vi "RIB Req - eSTOP 1.vi"(0 "Limits File Path":path, 5 "Results File Path":path, 11 "error in":errorcluster) -> (4 "Results Data Array":string[][](array[string]), 15 "error out":errorcluster)   [LabVIEW 2024]
doc: "Template test"
uses:
  <vilib>/addons/_JKI Toolkits/State Machine/_JKI_lib_State_Machine.llb/Select State(s)_err__jki_lib_state_machine.vi
  <vilib>/addons/_JKI Toolkits/State Machine/_JKI_lib_State_Machine.llb/Select State(s)_bool__jki_lib_state_machine.vi
  <vilib>/addons/_JKI Toolkits/State Machine/_JKI_lib_State_Machine.llb/Periodic Trigger__ogtk__JKI-SM__jki_lib_state_machine.vi
  <userlib>/_OpenG.lib/file/file.llb/Strip Path Extension - String__ogtk.vi
  <vilib>/Utility/file.llb/Read Delimited Spreadsheet (string).vi
  <userlib>/_OpenG.lib/file/file.llb/openg_file.lvlib
  <userlib>/_OpenG.lib/appcontrol/appcontrol.llb/openg_application_control.lvlib
  <userlib>/_OpenG.lib/time/time.llb/openg_time.lvlib
  <vilib>/Utility/file.llb/Write Delimited Spreadsheet (string).vi
panel:
  out "Wait for Start":bool
  out "Normal Operation":bool
  out "Wait - Reset":u32(slide)=1 scale=0.0..10.0
  in  "eSTOP 1 State Error Test":string
  in  "eSTOP 1 State Test":string
  in  "Read Start":string
  in  "Read Set":string
  out "Timeout - Error Test":dbl(slide) scale=0.0..3.0
  out "Timeout - Test":dbl(slide) scale=0.0..3.0
  out "eSTOP 1 Test":bool
  out "eSTOP 1 Error Test":bool
  in  "eSTOP 1 Error Test":string
  in  "eSTOP 1 Test":string
  in  "connection ID":refnum<k16>
  in  "handle out":u64
  in  "Exit":bool
  # "eSTOP 1 Test"
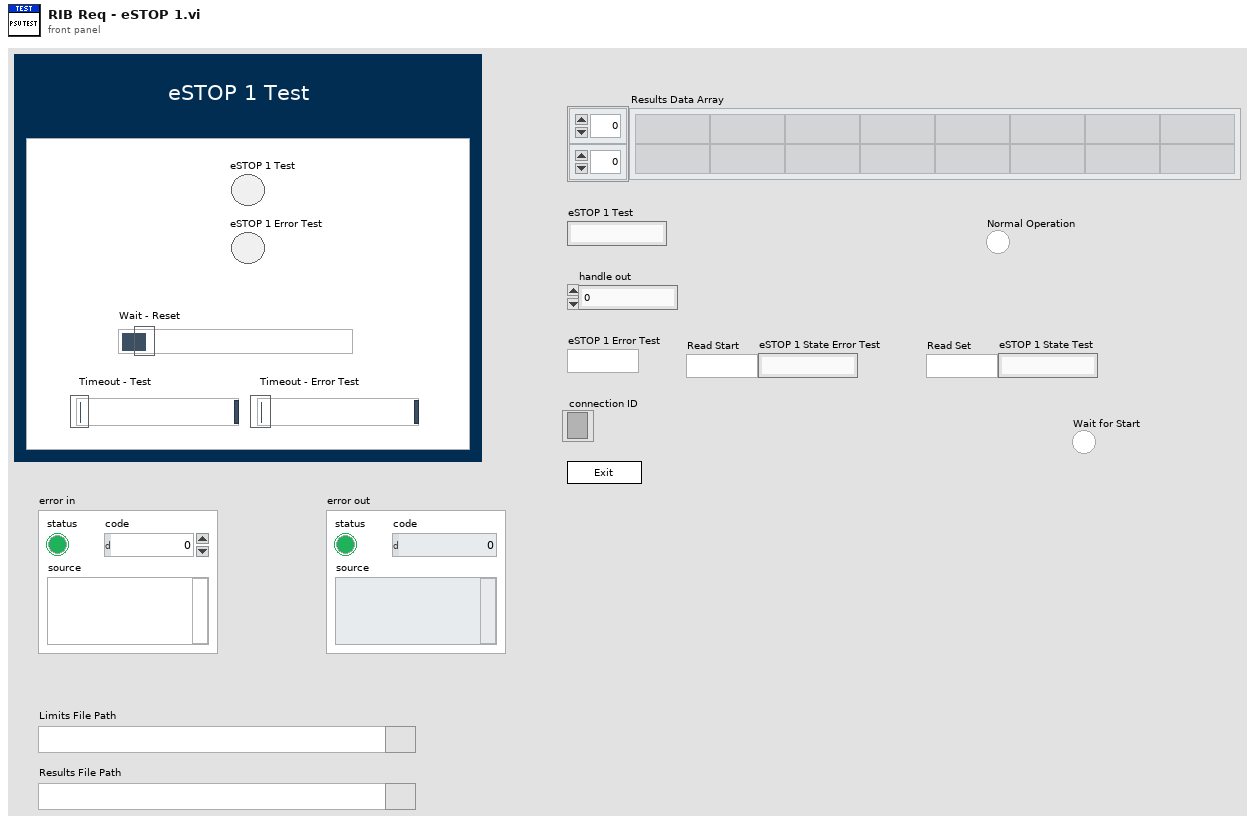
[diagram p1: front panel]
types:
  T1 = enum32{"Invalid", "Standard", "Closed", "Hidden", "Minimized", "Maximized"}
  T2 = enum32{"invalid app kind", "Development System", "Run Time System", "Student Edition", "Embedded LabVIEW", "Evaluation", "Custom"}
  T3 = typedef "FGV - Enum" = enum16{"Cleanup", "Get Data", "Open UDP", "Initialise DAQ", "Initialise I2C"}
  T4 = enum16{"Start Timer", "Get Time", "Pause", "Unpause"}
  T5 = cluster{"Core":cluster{"Current VI Reference":refnum<vi>, "Close Panel on Exit?":bool}, "Limits File Path":path, "Test Limits":string[][], "Results Data Array":string[][], "Results File Path":path, "Voltage":dbl, "connection ID":refnum<k16>, "handle out":u64, "eSTOP 1 Test":string, "eSTOP 1 Error Test":string, "Read Set":string, "Read Start ":string, "eSTOP 1 State Test":string, "eSTOP 1 State Error Test":string}
  T6 = cluster{"Current VI Reference":refnum<vi>, "Close Panel on Exit?":bool}
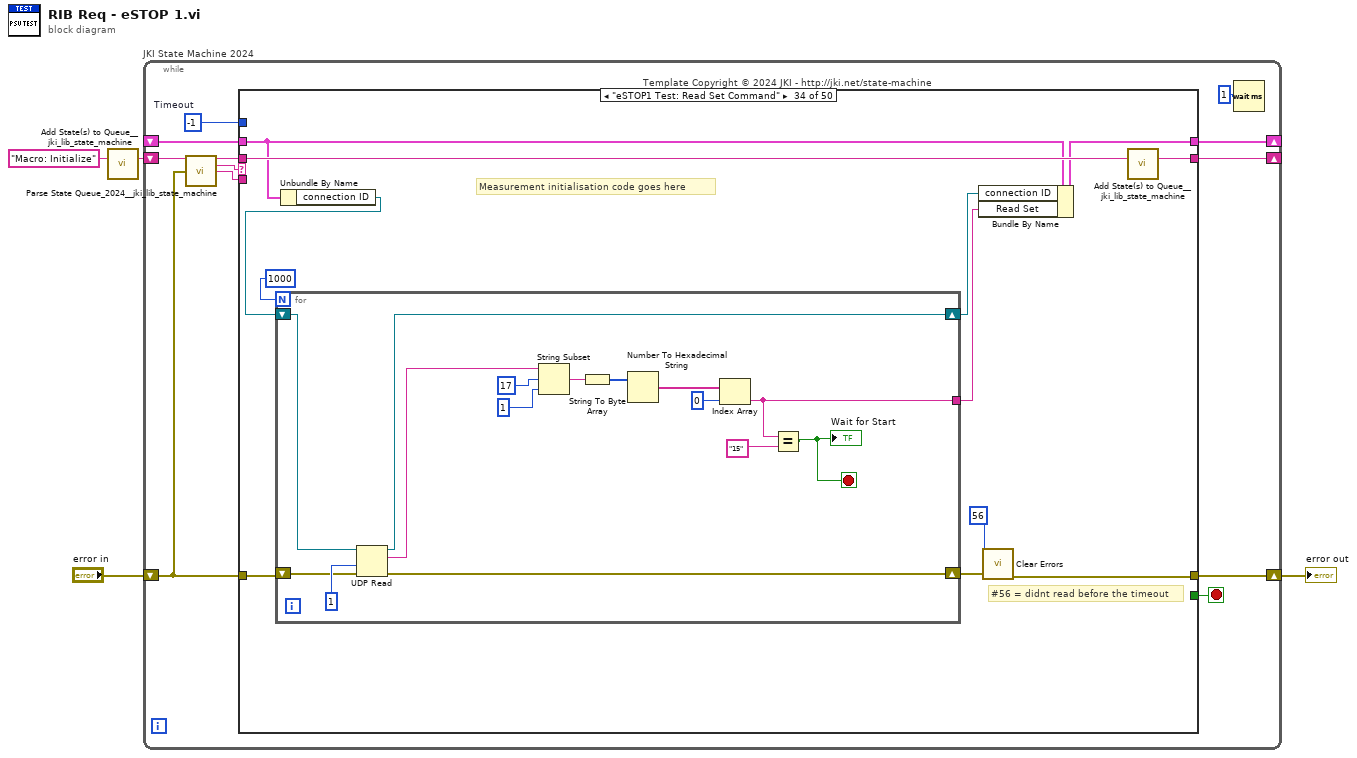
[diagram p0: block diagram]
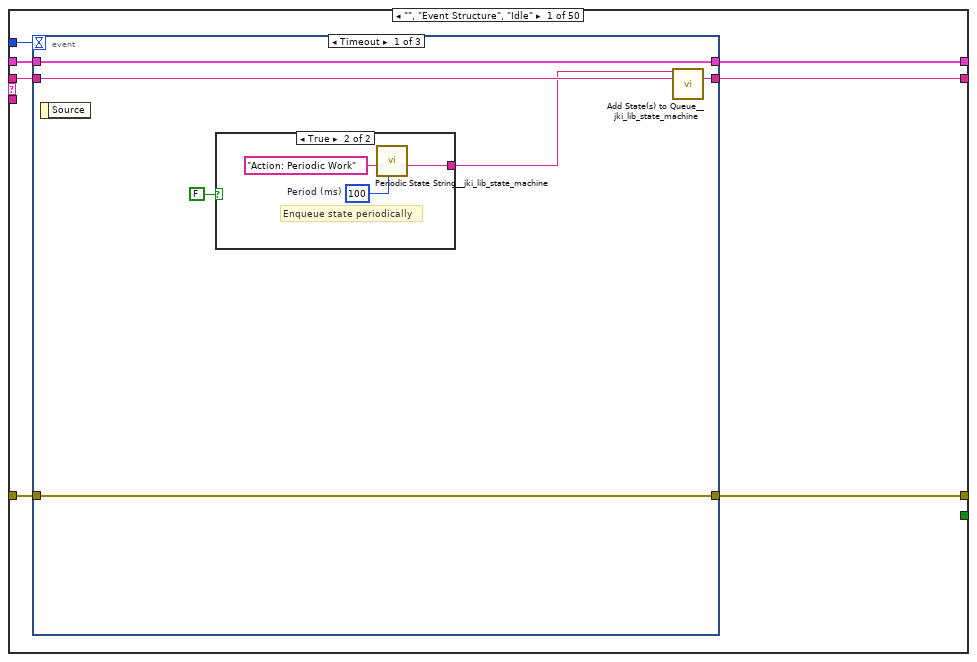
[diagram p2: hidden frame]
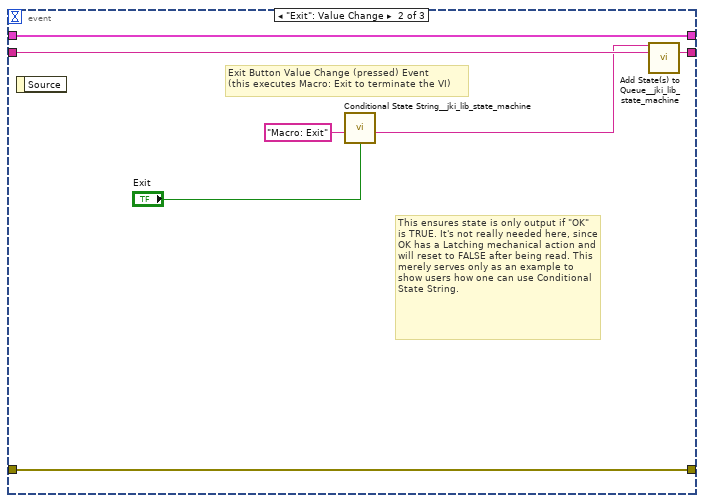
[diagram p4: hidden frame]
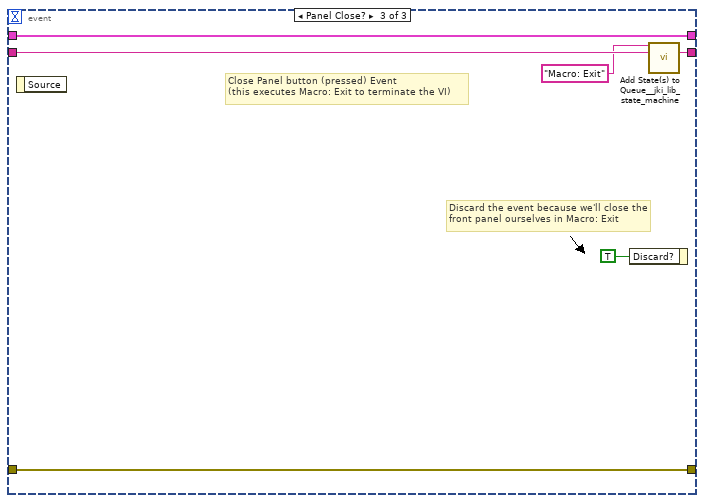
[diagram p5: hidden frame]
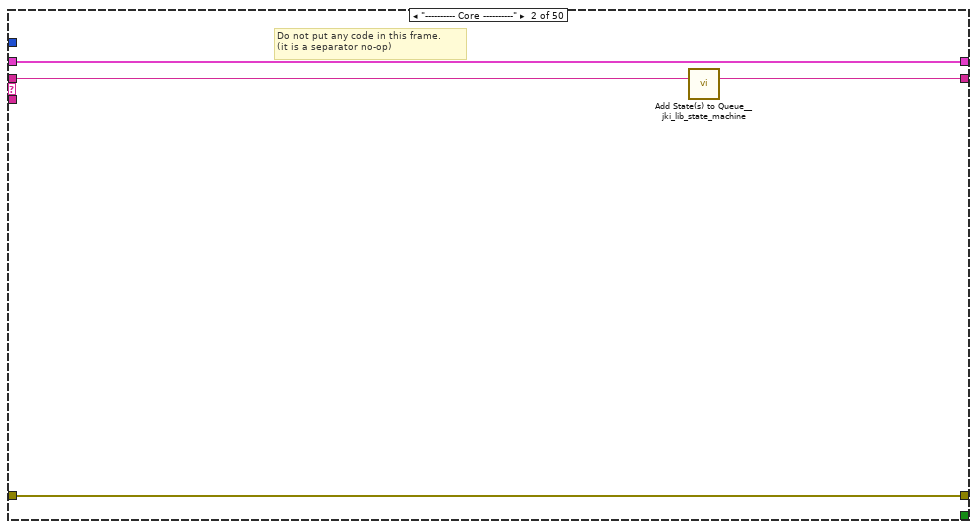
[diagram p6: hidden frame]
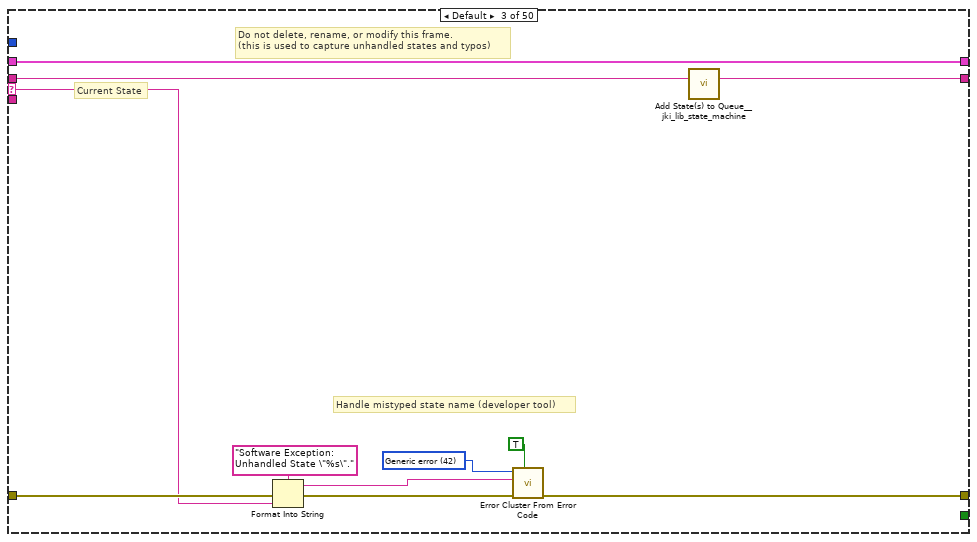
[diagram p7: hidden frame]
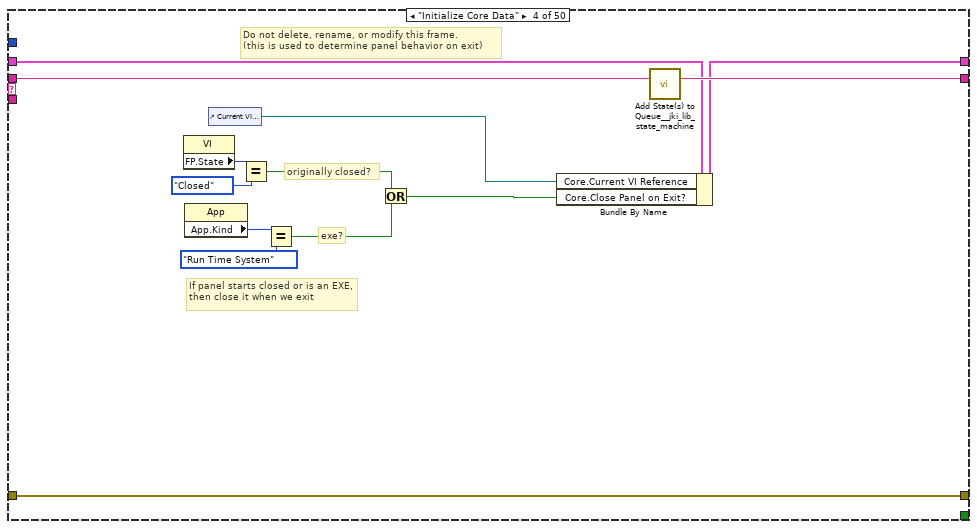
[diagram p8: hidden frame]
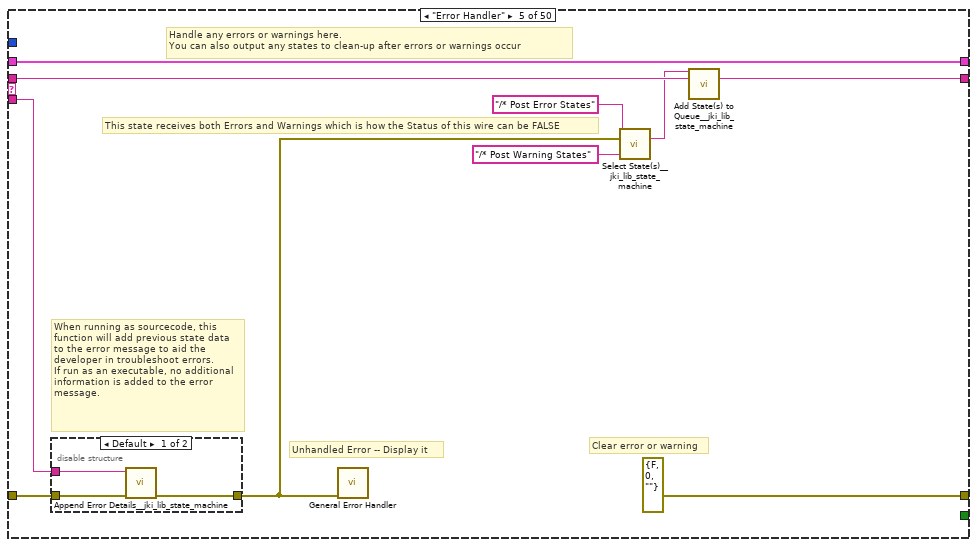
[diagram p9: hidden frame]
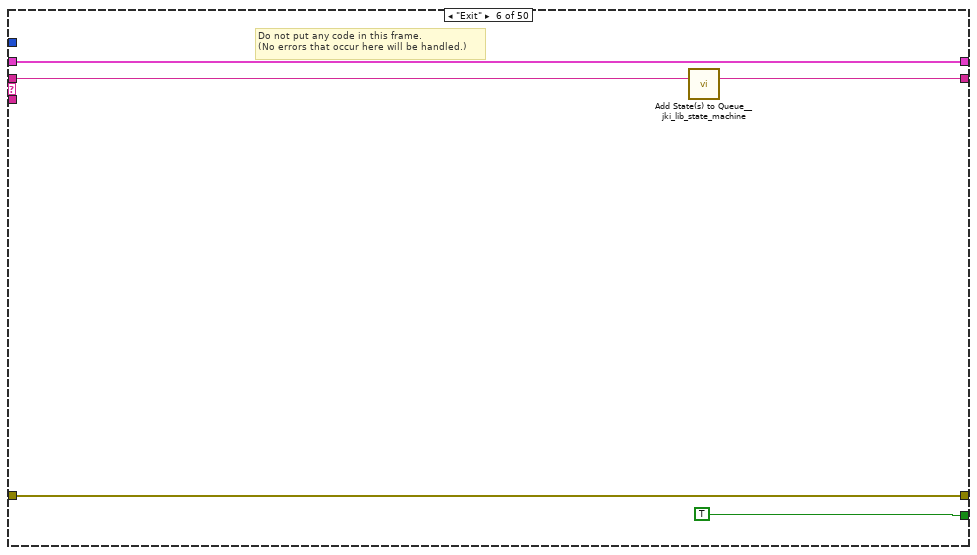
[diagram p11: hidden frame]
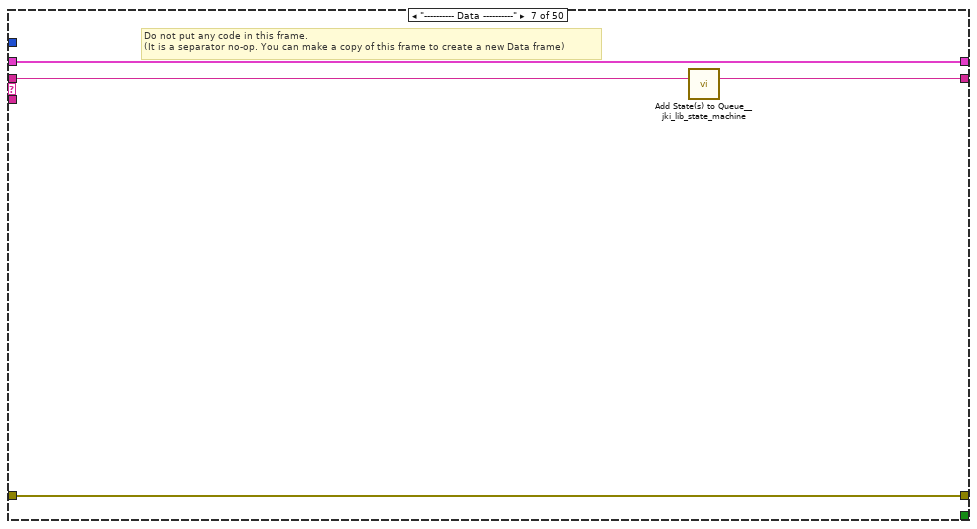
[diagram p12: hidden frame]
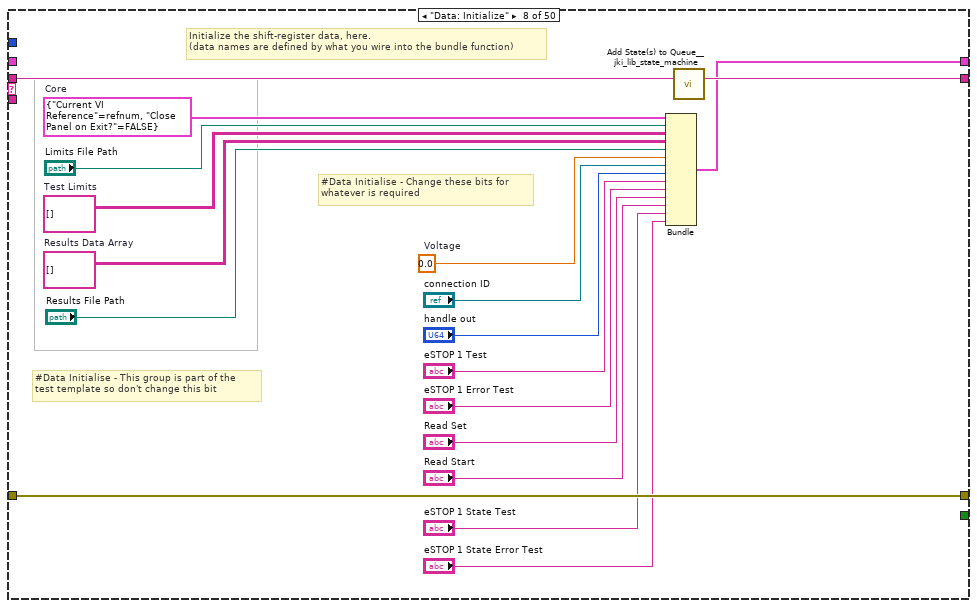
[diagram p13: hidden frame]
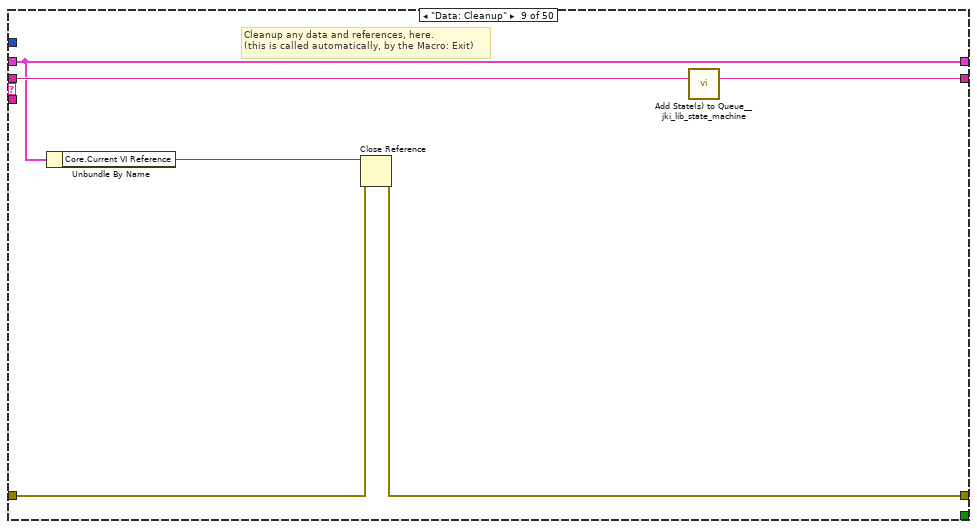
[diagram p14: hidden frame]
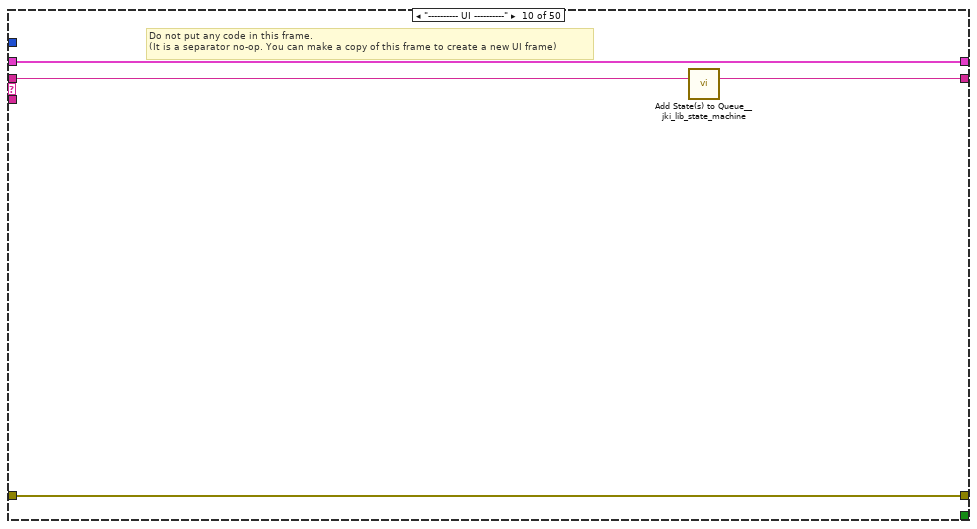
[diagram p15: hidden frame]
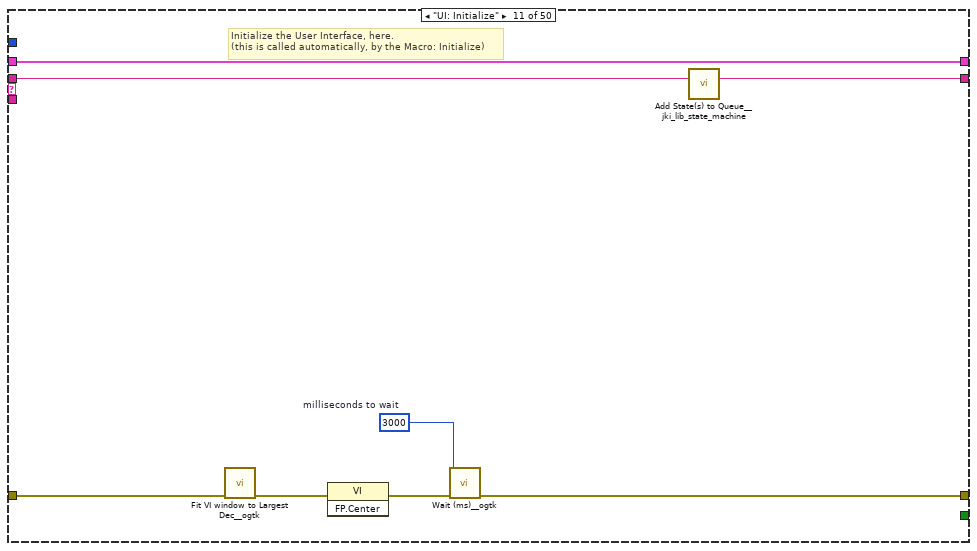
[diagram p16: hidden frame]
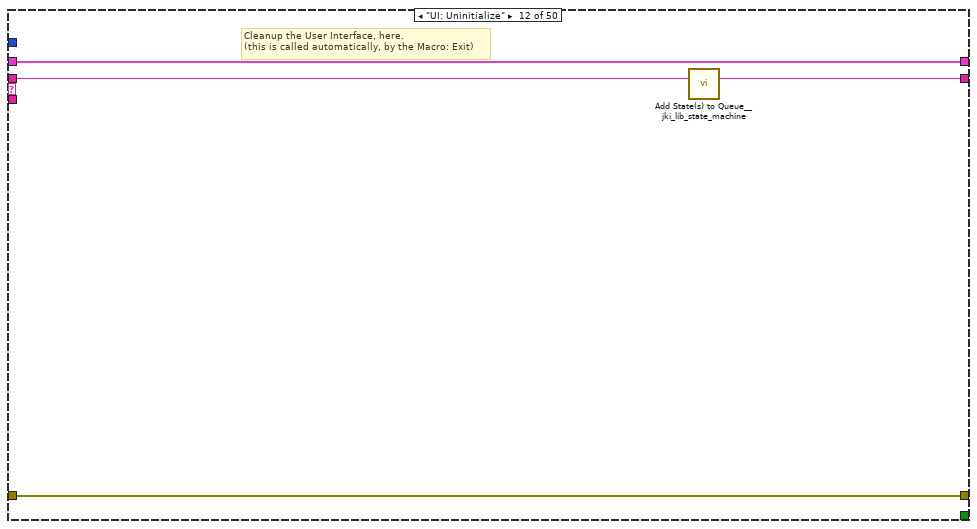
[diagram p17: hidden frame]
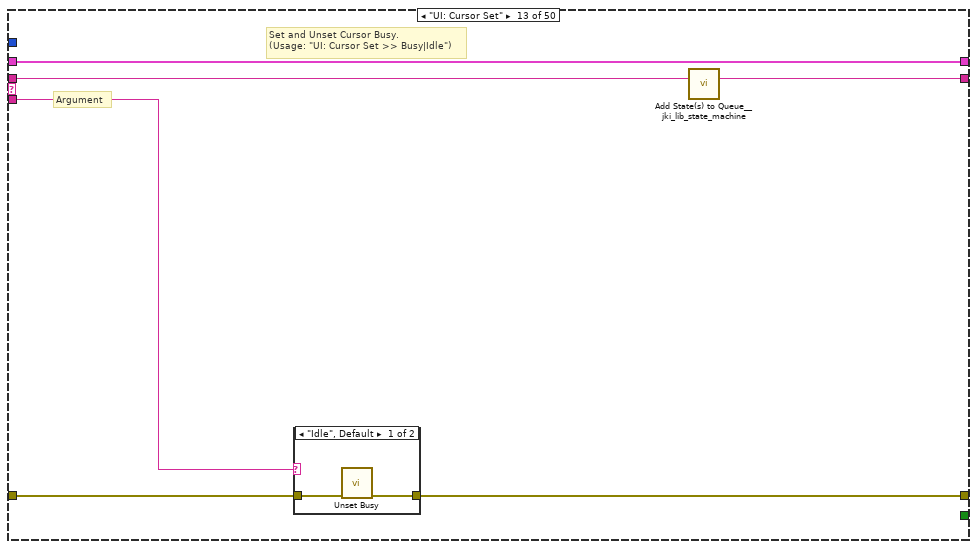
[diagram p18: hidden frame]
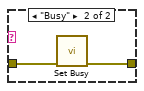
[diagram p19: hidden frame]
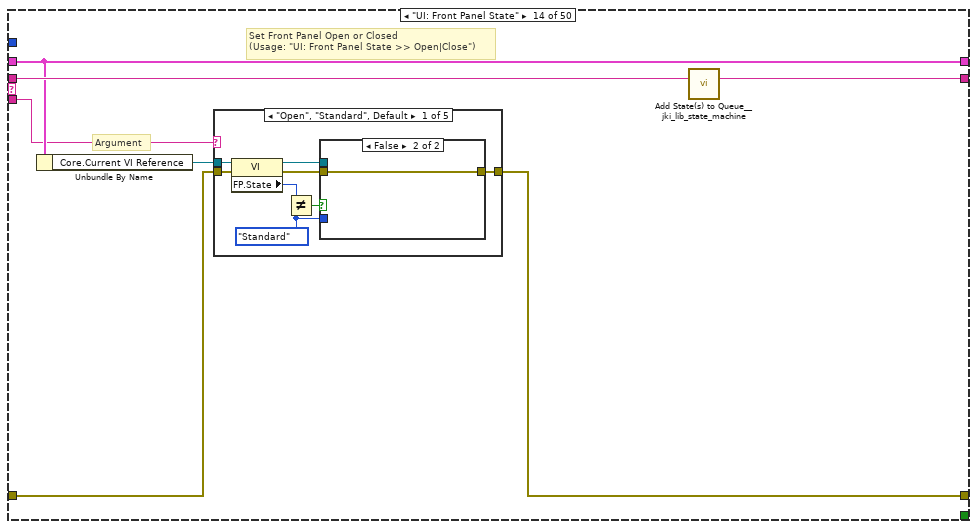
[diagram p20: hidden frame]
diagram:
  n1 = call <vilib>:"Add State(s) to Queue__jki_lib_state_machine.vi"("State(s) in (\"\")"="Macro: Initialize") -> ("States Out"=w4:string)  [unwired: 14 in]
  n2 = while "JKI State Machine 2024" {
    shift-right: [w9] -> _
    shift-left: _ -> [w8]
    shift-right: [w12] -> w1
    shift-left: "error in" -> [w6]
    shift-right: [w11] -> _
    shift-left: w4 -> [w13]
    stop <- w10 stop-if-true
    w7 = -1  # Timeout
    # "Template Copyright © 2024 JKI - http://jki.net/state-machine"
    n3 = call <vilib>:"Parse State Queue_2024__jki_lib_state_machine.vi"("State Queue"=w13, "Error In (no error)"=w6) -> ("Remaining States"=w15:string, "Current State"=w16:string, "Arguments"=w14:string)  [unwired: 11 in]
    n4 = case shown="\"eSTOP1 Test: Read Set Command\"" w16 {
      selector: w16 -> [_ _ w50 _ _ _ _ _ _ _ _ _ _ _ _ _ _ _ _ _ _ _ _ _ _ _ _ _ _ _ _ _ _ _ _ _ _ _ _ _ _ _ _ _ _ _ _ _ _ _]
      tunnel: w15 -> [w23 w49 w54 w73 w83 w92 w96 w114 w120 w124 w132 w136 w142 w153 w222 w227 w232 w237 w242 w251 w255 w268 w285 w298 w311 w324 w337 w350 w354 w363 w367 w376 w397 w409 w445 w457 w482 w491 w515 w539 w551 w560 w582 w603 w614 w624 w648 w672 w684 w693]
      tunnel: w14 -> [_ _ _ _ w78 _ _ _ _ _ _ _ w137 w147 _ _ _ _ _ _ _ _ _ _ _ _ _ _ _ _ _ _ _ _ _ _ _ _ _ _ _ _ _ _ _ _ _ _ _ _]
      tunnel: w8 -> [w21 w46 w52 w66 w80 w90 w93 _ w115 w121 w130 w134 w140 w149 w219 w224 w229 w234 w239 w249 w252 w258 w277 w290 w303 w316 w329 w342 w351 w359 w364 w374 w394 w406 w442 w454 w480 w485 w498 w522 w549 w553 w579 w600 w612 w618 w631 w655 w682 w686]
      tunnel: [w20 w47 w56 w70 errorcluster {"status"=FALSE, "code"=0, "source"=""} ("error out") w89 w94 w111 w116 w122 w128 w133 w138 w150 w220 w225 w230 w235 w240 w246 w253 w264 w282 w295 w308 w321 w334 w347 w352 w361 w365 w371 w378 w404 w426 w452 w473 w484 w496 w520 w543 w555 w563 w584 w605 w617 w629 w653 w676 w688] -> w12
      tunnel: w6 -> [w17 w47 w55 w70 w79 w89 w94 w111 w117 w122 w129 w133 w139 w151 w220 w225 w230 w235 w240 w246 w253 w263 w281 w294 w307 w320 w333 w346 w352 w360 w365 w372 w393 w400 w441 w446 w474 w488 w499 w523 w544 w554 w578 w599 w606 w621 w632 w656 w677 w687]
      tunnel: [w22 w48 w53 w72 w82 w91 w95 w113 w119 w123 w131 w135 w141 w152 w221 w226 w231 w236 w241 w250 w254 w267 w284 w297 w310 w323 w336 w349 w353 w362 w366 w375 w396 w408 w444 w456 w481 w490 w514 w538 w550 w559 w581 w602 w613 w623 w647 w671 w683 w692] -> w11
      tunnel: [_ _ _ _ _ TRUE _ _ _ _ _ _ _ _ _ _ _ _ _ _ _ _ _ _ _ _ _ _ _ _ _ _ _ _ _ _ _ _ _ _ _ _ _ _ _ _ _ _ _ _] -> w10
      tunnel: [w19 w46 w52 w71 w80 w90 w93 w112 w115 w121 w130 w134 w140 w149 w219 w224 w229 w234 w239 w249 w252 w257 w276 w289 w302 w315 w328 w341 w351 w359 w364 w373 w395 w407 w443 w455 w480 w483 w513 w537 w549 w552 w580 w601 w612 w616 w646 w670 w682 w685] -> w9
      tunnel: w7 -> [w18 _ _ _ _ _ _ _ _ _ _ _ _ _ _ _ _ _ _ _ _ _ _ _ _ _ _ _ _ _ _ _ _ _ _ _ _ _ _ _ _ _ _ _ _ _ _ _ _ _]
      frame "", "Event Structure", "Idle" {
        n5 = event shown="[0] Timeout" {
          selector: _ -> [_ _ _]
          dyn-events: _ -> [_ _ _]
          timeout: w18 -> [_ _ _]
          tunnel: w23 -> [w29 w39 w45]
          tunnel: [w28 w38 w44] -> w22
          tunnel: w21 -> [w26 w36 w42]
          tunnel: [w27 w37 w43] -> w20
          tunnel: w17 -> [w27 w37 w43]
          tunnel: [w26 w36 w42] -> w19
          event Timeout {
            n6 = event-data() -> ()  [unwired: 1 in, 1 out]
            n7 = case shown="True" FALSE {
              tunnel: [_ w32] -> w25
              frame False {
              }
              frame True {
                w30 = u32 100  # Period (ms)
                # "Enqueue state periodically"
                n8 = call <vilib>:"Periodic State String__jki_lib_state_machine.vi"("Period (ms)"=w30, "State"="Action: Periodic Work") -> ("State Out"=w32:string)  [unwired: 9 in]
              }
            }
            n9 = call <vilib>:"Add State(s) to Queue__jki_lib_state_machine.vi"("State(s) in Front (\"\")"=w25, "State(s) in (\"\")"=w29) -> ("States Out"=w28:string)  [unwired: 13 in]
          }
          event "Exit": Value Change {
            # "This ensures state is only output if \"OK\" is TRUE. It's not really needed here, since OK has a Latching mechanical action and will reset to FALSE after being read. This merely serves only as an example to show users how one can use Conditional State String."
            # "Exit Button Value Change (pressed) Event\n(this executes Macro: Exit to terminate the VI)"
            n10 = event-data() -> ()  [unwired: 1 in, 1 out]
            n11 = call <vilib>:"Conditional State String__jki_lib_state_machine.vi"("Do State(s)?"="Exit", "State"="Macro: Exit") -> ("State Out"=w33:string)  [unwired: 7 in]
            n12 = call <vilib>:"Add State(s) to Queue__jki_lib_state_machine.vi"("State(s) in Front (\"\")"=w33, "State(s) in (\"\")"=w39) -> ("States Out"=w38:string)  [unwired: 13 in]
          }
          event Panel Close? {
            # "Discard the event because we'll close the front panel ourselves in Macro: Exit"
            # "Close Panel button (pressed) Event\n(this executes Macro: Exit to terminate the VI)"
            n13 = event-data() -> ()  [unwired: 1 in, 1 out]
            n14 = event-data("Discard?"=TRUE) -> ()  [unwired: 1 in, 1 out]
            n15 = call <vilib>:"Add State(s) to Queue__jki_lib_state_machine.vi"("State(s) in Front (\"\")"="Macro: Exit", "State(s) in (\"\")"=w45) -> ("States Out"=w44:string)  [unwired: 13 in]
          }
        }
      }
      frame "---------- Core ----------" {
        # "Do not put any code in this frame.\n(it is a separator no-op)"
        n16 = call <vilib>:"Add State(s) to Queue__jki_lib_state_machine.vi"("State(s) in (\"\")"=w49) -> ("States Out"=w48:string)  [unwired: 14 in]
      }
      frame Default {
        w59 = 42 items=["No error", "Argument error", "Memory is full", "Out of zone", "End of file", "File already open", "Generic file I/O error", "File not found", "File permission error", "Disk is full", "Duplicate path", "Too many files open", "System feature not enabled", "Resource file not found", "Cannot add resource", "Resource not found", "Image not found", "Image memory error", "Pen does not exist", "Config type invalid", "Config token not found", "Config parse error", "Config memory error", "Bad external code format", "Bad external code offset", "External code not present", "Null window", "Destroy window error", "Null menu", "Print aborted", "Bad print record", "Print driver error", "Windows error during printing", "Memory error during printing", "Print dialog error", "Generic print error", "Invalid device refnum", "Device not found", "Device parameter error", "Device unit error", "Cannot open device", "Device call aborted", "Generic error", "Cancelled by user", "Object ID too low", "Object ID too high", "Object not in heap", "Unknown heap", "Unknown object (invalid DefProc)", "Unknown object (DefProc not in table)", "Message out of range", "Invalid (null) method", "Unknown message", "Manager call not supported", "Bad address", "Network operation in progress", "Network operation timed out", "Connection is busy", "Network attribute not supported", "Network error", "Address in use", "System out of memory", "Connection aborted", "Connection refused", "Not connected", "Already connected", "Connection closed", "Initialization error (interapplication manager)", "Bad occurrence", "Wait on unbound occurrence handler", "Occurrence queue overflow", "Datalog type conflict", "Unused", "Unrecognized type (interapplication manager)", "Memory corrupt", "Failed to make temporary DLL", "Old CIN version", "Drag socket not found", "Failed to load drop-object", "Failed to register OLE object", "Failed to release OLE object", "Format specifier type mismatch", "Unknown format specifier", "Too few format specifiers", "Too many format specifiers", "Scan failed", "Newer CIN version", "Error converting to variant", "Runtime menu error", "Password tampered", "Variant attribute not found", "Incompatible variant data type", "Event data is not available", "Event Store is not present", "Occurrence is not found", "Event Queue is not created", "Event info is not available", "Refnum passed is NULL", "Error retrieving Class GUID", "Error retrieving CoClass GUID", "Error retrieving TypeLib GUID.", "Bad built application magic bytes.", "Specific driver is different from the specific driver associated with the Logical Name.", "There is no session opened to the class driver.", "Max Error", "MAX - Error with config objects", "MAX - Error loading configuration", "MAX - Group not supported"]
        # "Current State"
        # "Do not delete, rename, or modify this frame.\n(this is used to capture unhandled states and typos)"
        # "Handle mistyped state name (developer tool)"
        n17 = Format Into String(format string="Software Exception: Unhandled State \"%s\"." ("message"), error in=w55, w50) -> (resulting string=w58:string, error out=w57:errorcluster)  [unwired: 1 in]
        n18 = call <vilib>:"Error Cluster From Error Code.vi"("show call chain? (False)"=TRUE, "error in (no error)"=w57, "error message (\"\")"=w58, "error code (0)"=w59) -> ("error out"=w56:errorcluster)  [unwired: 5 in]
        n19 = call <vilib>:"Add State(s) to Queue__jki_lib_state_machine.vi"("State(s) in (\"\")"=w54) -> ("States Out"=w53:string)  [unwired: 14 in]
      }
      frame "Initialize Core Data" {
        # "Do not delete, rename, or modify this frame.\n(this is used to determine panel behavior on exit)"
        # "originally closed?"
        # "exe?"
        # "If panel starts closed or is an EXE, then close it when we exit"
        n20 = property class="VI"() -> ("FP.State"=w63:T1)  [unwired: 2 in, 2 out]
        n21 = property class="App"() -> ("App.Kind"=w69:T2)  [unwired: 2 in, 2 out]
        n22 = control-ref of="Current VI Reference"() -> (w64:refnum<vi>)
        n23 = Equal?(x=w63, y=T1."Closed" ("Front Panel Window:State")) -> (x = y?=w61:bool)
        n24 = Equal?(x=w69, y=T2."Run Time System" ("Application:Kind")) -> (x = y?=w67:bool)
        n25 = Or(x=w61, y=w67) -> (x .or. y?=w65:bool)
        n26 = Bundle By Name(cluster=w66, "Core.Current VI Reference"=w64, "Core.Close Panel on Exit?"=w65) -> (w71:T5)
        n27 = call <vilib>:"Add State(s) to Queue__jki_lib_state_machine.vi"("State(s) in (\"\")"=w73) -> ("States Out"=w72:string)  [unwired: 14 in]
      }
      frame "Error Handler" {
        # "When running as sourcecode, this function will add previous state data to the error message to aid the developer in troubleshoot errors.\nIf run as an executable, no additional information is added to the error message."
        # "This state receives both Errors and Warnings which is how the Status of this wire can be FALSE"
        # "Unhandled Error -- Display it"
        # "Handle any errors or warnings here.\nYou can also output any states to clean-up after errors or warnings occur"
        # "Clear error or warning"
        n28 = disable-structure shown="Default" {
          disable-tunnel: w79 -> [w86 w87]
          disable-tunnel: w78 -> [w85 _]
          disable-tunnel: [w84 w87] -> w77
          frame condition #0 (active) {
            n29 = call <vilib>:"Append Error Details__jki_lib_state_machine.vi"("error in (no error)"=w86, "Previous State and Argument(s)"=w85) -> ("error out"=w84:errorcluster)  [unwired: 9 in]
          }
          frame condition #1 {
          }
        }
        n30 = call <vilib>:"General Error Handler.vi"("error in (no error)"=w77) -> ()  [unwired: 10 in, 5 out]
        n31 = call-poly <vilib>:"Select State(s)__jki_lib_state_machine.vi"("State(s) if True (\"\")"="/* Post Error States", "Select"=w77, "State(s) if False (\"\")"="/* Post Warning States") -> ("States Out"=w75:string)  [unwired: 12 in]
        n32 = call <vilib>:"Add State(s) to Queue__jki_lib_state_machine.vi"("State(s) in Front (\"\")"=w75, "State(s) in (\"\")"=w83) -> ("States Out"=w82:string)  [unwired: 13 in]
      }
      frame "Exit" {
        # "Do not put any code in this frame.\n(No errors that occur here will be handled.)"
        n33 = call <vilib>:"Add State(s) to Queue__jki_lib_state_machine.vi"("State(s) in (\"\")"=w92) -> ("States Out"=w91:string)  [unwired: 14 in]
      }
      frame "---------- Data ----------" {
        # "Do not put any code in this frame.\n(It is a separator no-op. You can make a copy of this frame to create a new Data frame)"
        n34 = call <vilib>:"Add State(s) to Queue__jki_lib_state_machine.vi"("State(s) in (\"\")"=w96) -> ("States Out"=w95:string)  [unwired: 14 in]
      }
      frame "Data: Initialize" {
        w105 = 0.0  # Voltage
        w107 = string[][] []  # Results Data Array
        w108 = string[][] []  # Test Limits
        w110 = T6 {"Current VI Reference"=refnum, "Close Panel on Exit?"=FALSE}  # Core
        # "#Data Initialise - Change these bits for\nwhatever is required"
        # "#Data Initialise - This group is part of the\ntest template so don't change this bit"
        # "Initialize the shift-register data, here.\n(data names are defined by what you wire into the bundle function)"
        n35 = Bundle("Core"=w110, "Limits File Path"="Limits File Path", "Test Limits"=w108, "Results Data Array"=w107, "Results File Path"="Results File Path", "Voltage"=w105, "connection ID"="connection ID", "handle out"="handle out", "eSTOP 1 Test"="eSTOP 1 Test", "eSTOP 1 Error Test"="eSTOP 1 Error Test", "Read Set"="Read Set", "Read Start"="Read Start", "eSTOP 1 State Test"="eSTOP 1 State Test", "eSTOP 1 State Error Test"="eSTOP 1 State Error Test") -> (w112:T5)  [unwired: 1 in]
        n36 = call <vilib>:"Add State(s) to Queue__jki_lib_state_machine.vi"("State(s) in (\"\")"=w114) -> ("States Out"=w113:string)  [unwired: 14 in]
      }
      frame "Data: Cleanup" {
        # "Cleanup any data and references, here.\n(this is called automatically, by the Macro: Exit)"
        n37 = Unbundle By Name(w115) -> ("Core.Current VI Reference"=w118:refnum<vi>)
        n38 = Close Reference(reference=w118, error in (no error)=w117) -> (error out=w116:errorcluster)
        n39 = call <vilib>:"Add State(s) to Queue__jki_lib_state_machine.vi"("State(s) in (\"\")"=w120) -> ("States Out"=w119:string)  [unwired: 14 in]
      }
      frame "---------- UI ----------" {
        # "Do not put any code in this frame.\n(It is a separator no-op. You can make a copy of this frame to create a new UI frame)"
        n40 = call <vilib>:"Add State(s) to Queue__jki_lib_state_machine.vi"("State(s) in (\"\")"=w124) -> ("States Out"=w123:string)  [unwired: 14 in]
      }
      frame "UI: Initialize" {
        w127 = u32 3000  # milliseconds to wait
        # "Initialize the User Interface, here.\n(this is called automatically, by the Macro: Initialize)"
        n41 = call <userlib>:"Fit VI window to Largest Dec__ogtk.vi"("error in (no error)"=w129) -> ("error out"=w125:errorcluster)  [unwired: 5 in, 1 out]
        n42 = invoke class="VI" method="FP.Center"(error in=w125) -> (error out=w126:errorcluster)  [unwired: 2 in, 2 out]
        n43 = call <userlib>:"Wait (ms)__ogtk.vi"("error in (no error)"=w126, "milliseconds to wait"=w127) -> ("error out"=w128:errorcluster)  [unwired: 8 in, 1 out]
        n44 = call <vilib>:"Add State(s) to Queue__jki_lib_state_machine.vi"("State(s) in (\"\")"=w132) -> ("States Out"=w131:string)  [unwired: 14 in]
      }
      frame "UI: Uninitialize" {
        # "Cleanup the User Interface, here.\n(this is called automatically, by the Macro: Exit)"
        n45 = call <vilib>:"Add State(s) to Queue__jki_lib_state_machine.vi"("State(s) in (\"\")"=w136) -> ("States Out"=w135:string)  [unwired: 14 in]
      }
      frame "UI: Cursor Set" {
        # "Argument"
        # "Set and Unset Cursor Busy.\n(Usage: \"UI: Cursor Set >> Busy|Idle\")"
        n46 = case shown="\"Idle\", Default" w137 {
          tunnel: w139 -> [w144 w146]
          tunnel: [w143 w145] -> w138
          frame "Idle", Default {
            n47 = call <vilib>:"Unset Busy.vi"("error in (no error)"=w144) -> ("error out"=w143:errorcluster)  [unwired: 10 in]
          }
          frame "Busy" {
            n48 = call <vilib>:"Set Busy.vi"("error in (no error)"=w146) -> ("error out"=w145:errorcluster)  [unwired: 9 in, 1 out]
          }
        }
        n49 = call <vilib>:"Add State(s) to Queue__jki_lib_state_machine.vi"("State(s) in (\"\")"=w142) -> ("States Out"=w141:string)  [unwired: 14 in]
      }
      frame "UI: Front Panel State" {
        # "Argument"
        # "Set Front Panel Open or Closed\n(Usage: \"UI: Front Panel State >> Open|Close\")"
        n50 = Unbundle By Name(w149) -> ("Core.Current VI Reference"=w148:refnum<vi>)
        n51 = case shown="\"Open\", \"Standard\", Default" w147 {
          tunnel: w151 -> [w159 w174 w185 w198 w211]
          tunnel: [w161 w175 w187 w200 w213] -> w150
          tunnel: w148 -> [w160 w172 w186 w199 w212]
          frame "Open", "Standard", Default {
            w154 = T1."Standard" ("State")
            n52 = property class="VI"(reference=w160, error in=w159) -> (reference out=w157:refnum<vi>, error out=w158:errorcluster, "FP.State"=w156:T1)
            n53 = Not Equal?(x=w156, y=w154) -> (x != y?=w155:bool)
            n54 = case shown="False" w155 {
              tunnel: [w165 w167] -> w161
              tunnel: w158 -> [w164 w167]
              tunnel: w157 -> [w163 _]
              tunnel: w154 -> [w162 _]
              frame True {
                n55 = invoke class="VI" method="FP.Open"(reference=w163, error in=w164, "Activate"=TRUE, "State"=w162) -> (error out=w165:errorcluster)  [unwired: 1 in, 4 out]
              }
              frame False {
              }
            }
          }
          frame "Close", "Closed" {
            n56 = property class="VI"(reference=w172, error in=w174) -> (reference out=w171:refnum<vi>, error out=w173:errorcluster, "FP.State"=w169:T1)
            n57 = Not Equal?(x=w169, y=T1."Closed" ("Front Panel Window:State")) -> (x != y?=w168:bool)
            n58 = case shown="True" w168 {
              tunnel: [w176 w179] -> w175
              tunnel: w173 -> [w176 w178]
              tunnel: w171 -> [_ w177]
              frame False {
              }
              frame True {
                n59 = invoke class="VI" method="FP.Close"(reference=w177, error in=w178) -> (error out=w179:errorcluster)  [unwired: 1 in, 2 out]
              }
            }
          }
          frame "Hidden", "Hide" {
            w180 = T1."Hidden" ("State")
            n60 = property class="VI"(reference=w186, error in=w185) -> (reference out=w183:refnum<vi>, error out=w184:errorcluster, "FP.State"=w182:T1)
            n61 = Not Equal?(x=w182, y=w180) -> (x != y?=w181:bool)
            n62 = case shown="True" w181 {
              tunnel: [w191 w192] -> w187
              tunnel: w184 -> [w190 w192]
              tunnel: w183 -> [w189 _]
              tunnel: w180 -> [w188 _]
              frame True {
                n63 = invoke class="VI" method="FP.Open"(reference=w189, error in=w190, "State"=w188) -> (error out=w191:errorcluster)  [unwired: 2 in, 4 out]
              }
              frame False {
              }
            }
          }
          frame "Minimize", "Minimized" {
            w193 = T1."Minimized" ("State")
            n64 = property class="VI"(reference=w199, error in=w198) -> (reference out=w196:refnum<vi>, error out=w197:errorcluster, "FP.State"=w195:T1)
            n65 = Not Equal?(x=w195, y=w193) -> (x != y?=w194:bool)
            n66 = case shown="True" w194 {
              tunnel: [w204 w205] -> w200
              tunnel: w197 -> [w203 w205]
              tunnel: w196 -> [w202 _]
              tunnel: w193 -> [w201 _]
              frame True {
                n67 = invoke class="VI" method="FP.Open"(reference=w202, error in=w203, "State"=w201) -> (error out=w204:errorcluster)  [unwired: 2 in, 4 out]
              }
              frame False {
              }
            }
          }
          frame "Maximize", "Maximized" {
            w206 = T1."Maximized" ("State")
            n68 = property class="VI"(reference=w212, error in=w211) -> (reference out=w209:refnum<vi>, error out=w210:errorcluster, "FP.State"=w208:T1)
            n69 = Not Equal?(x=w208, y=w206) -> (x != y?=w207:bool)
            n70 = case shown="True" w207 {
              tunnel: [w217 w218] -> w213
              tunnel: w210 -> [w216 w218]
              tunnel: w209 -> [w215 _]
              tunnel: w206 -> [w214 _]
              frame True {
                n71 = invoke class="VI" method="FP.Open"(reference=w215, error in=w216, "State"=w214) -> (error out=w217:errorcluster)  [unwired: 2 in, 4 out]
              }
              frame False {
              }
            }
          }
        }
        n72 = call <vilib>:"Add State(s) to Queue__jki_lib_state_machine.vi"("State(s) in (\"\")"=w153) -> ("States Out"=w152:string)  [unwired: 14 in]
      }
      frame "---------- Macro ----------" {
        # "Do not put any code in this frame.\n(It is a separator no-op. You can make a copy of this frame to create a new Macro frame)"
        n73 = call <vilib>:"Add State(s) to Queue__jki_lib_state_machine.vi"("State(s) in (\"\")"=w222) -> ("States Out"=w221:string)  [unwired: 14 in]
      }
      frame "Macro: Initialize" {
        # "Initialization Macro\n(This is called once, when the VI starts)"
        n74 = call <vilib>:"Add State(s) to Queue__jki_lib_state_machine.vi"("State(s) in Front (\"\")"="Data: Initialize\nInitialize Core Data\nUI: Initialize\nUI: Front Panel State >> Open\neSTOP1 Test: Initialise\nMacro: Test", "State(s) in (\"\")"=w227) -> ("States Out"=w226:string)  [unwired: 13 in]
      }
      frame "Macro: Test" {
        # "#Test Macro - Add the sequence \nfor measurments and limits testing here"
        n75 = call <vilib>:"Add State(s) to Queue__jki_lib_state_machine.vi"("State(s) in Front (\"\")"="Limits Test: Read Limits File\neSTOP1 Test: Initialise\neSTOP1 Test: Set Command\neSTOP1 Test: Read Set Command\neSTOP1 Test: Start Command\neSTOP1 Test: Read Start Command\neSTOP1 Test: Start Timer\neSTOP1 Test: I2C Measurment\neSTOP1 Test: UDP Read", "State(s) in (\"\")"=w232) -> ("States Out"=w231:string)  [unwired: 13 in]
      }
      frame "Macro: Test (Error)" {
        # "#Test Macro - Add the sequence \nfor measurments and limits testing here"
        n76 = call <vilib>:"Add State(s) to Queue__jki_lib_state_machine.vi"("State(s) in Front (\"\")"="eSTOP1 Test: Reset\neSTOP1 Test: Set Command (Error)\neSTOP1 Test: Start Command (Error)\neSTOP1 Test: Start Timer (Error)", "State(s) in (\"\")"=w237) -> ("States Out"=w236:string)  [unwired: 13 in]
      }
      frame "Macro: Limits" {
        # "Do not put any code in this frame.\n(It is a separator no-op. You can make a copy of this frame to create a new Macro frame)"
        n77 = call <vilib>:"Add State(s) to Queue__jki_lib_state_machine.vi"("State(s) in Front (\"\")"="Limits Test: eSTOP 1 Test\nLimits Test: eSTOP 1 Error Test\nLimits Test: Read Set\nLimits Test: Read Start\nLimits Test: eSTOP 1 State Error Test\nLimits Test: eSTOP 1 State Test\nResults Data: Write Results Data\nMacro: Exit", "State(s) in (\"\")"=w242) -> ("States Out"=w241:string)  [unwired: 13 in]
      }
      frame "Macro: Exit" {
        # "Exit Macro\n(This is called once, when the VI exits)"
        n78 = Unbundle By Name(w249) -> ("Core.Close Panel on Exit?"=w244:bool)
        n79 = call <vilib>:"Conditional State String__jki_lib_state_machine.vi"("Do State(s)?"=w244, "State"="UI: Front Panel State >> Close") -> ("State Out"=w243:string)  [unwired: 7 in]
        n80 = call <vilib>:"Add State(s) to Queue__jki_lib_state_machine.vi"("State(s) in (\"\")"=w243, "State(s) at Back (\"\")"="eSTOP1 Test: Cleanup\nUI: Uninitialize\nData: Cleanup\nExit") -> ("States Out"=w247:string)  [unwired: 13 in]
        n81 = call <vilib>:"Add State(s) to Queue__jki_lib_state_machine.vi"("State(s) in Front (\"\")"=w247, "State(s) in (\"\")"=w251) -> ("States Out"=w250:string)  [unwired: 13 in]
      }
      frame "---------- Limits Test ----------" {
        # "Template Separator\n(You can make a copy of, or modify, this frame)"
        n82 = call <vilib>:"Add State(s) to Queue__jki_lib_state_machine.vi"("State(s) in (\"\")"=w255) -> ("States Out"=w254:string)  [unwired: 14 in]
      }
      frame "Limits Test: Read Limits File" {
        w261 = ","  # delimiter (\t)
        n83 = Unbundle By Name(w258) -> ("Limits File Path"=w262:path)
        n84 = Current VI's Path "Test Case Path"() -> (path=w266:path)
        n85 = call-poly <vilib>:"Read Delimited Spreadsheet.vi"("file path (dialog if empty)"=w262, "error in (no error)"=w263, "delimiter (\\t)"=w261) -> ("all rows"=w259:string[][], "error out"=w264:errorcluster)  [unwired: 7 in, 4 out]
        n86 = Strip Path(path=w266) -> (name=w265:string)  [unwired: 1 out]
        n87 = call-poly <userlib>:"Strip Path Extension__ogtk.vi"("path"=w265) -> ("root"=w260:string)  [unwired: 1 out]
        n88 = for {
          tunnel: w260 -> [w272]
          tunnel: w259 -> [w270] mode=indexing
          tunnel: [w270] -> w256 mode=indexing if=w269
          n89 = Index Array(array=w270) -> (element=w271:string)  [unwired: 1 in]
          n90 = Equal?(x=w272, y=w271) -> (x = y?=w269:bool)
        }
        n91 = Bundle By Name(cluster=w258, "Test Limits"=w256) -> (w257:T5)
        n92 = call <vilib>:"Add State(s) to Queue__jki_lib_state_machine.vi"("State(s) in (\"\")"=w268) -> ("States Out"=w267:string)  [unwired: 14 in]
      }
      frame "Limits Test: eSTOP 1 Test" {
        w278 = "eSTOP 1 Test"  # Sub Test Name
        # "Equal to F1?"
        # "#Limits Testing - Add the sub test name for\ntest included in limits file"
        n93 = Unbundle By Name(w277) -> ("Test Limits"=w279:string[][], "eSTOP 1 Test"=w283:string)
        n94 = Unbundle By Name(w277) -> ("Results Data Array"=w275:string[][])
        n95 = To Variant(anything=w283) -> (Variant=w280:variant)
        n96 = call "Process Results.vi"("error in (no error)"=w281, "Measurement"=w280, "Test Limits"=w279, "Sub Test Name"=w278) -> ("error out"=w282:errorcluster, "Results Data"=w274:string[])  [unwired: 6 in]
        n97 = Build Array (concatenate)(w275, w274) -> (w273:string[][])
        n98 = Bundle By Name(cluster=w277, "Results Data Array"=w273) -> (w276:T5)
        n99 = call <vilib>:"Add State(s) to Queue__jki_lib_state_machine.vi"("State(s) in (\"\")"=w285) -> ("States Out"=w284:string)  [unwired: 14 in]
      }
      frame "Limits Test: eSTOP 1 State Test" {
        w291 = "eSTOP 1 State Test"  # Sub Test Name
        # "Equal to F1?"
        # "#Limits Testing - Add the sub test name for\ntest included in limits file"
        n100 = Unbundle By Name(w290) -> ("Test Limits"=w292:string[][], "eSTOP 1 State Test"=w296:string)
        n101 = Unbundle By Name(w290) -> ("Results Data Array"=w288:string[][])
        n102 = To Variant(anything=w296) -> (Variant=w293:variant)
        n103 = call "Process Results.vi"("error in (no error)"=w294, "Measurement"=w293, "Test Limits"=w292, "Sub Test Name"=w291) -> ("error out"=w295:errorcluster, "Results Data"=w287:string[])  [unwired: 6 in]
        n104 = Build Array (concatenate)(w288, w287) -> (w286:string[][])
        n105 = Bundle By Name(cluster=w290, "Results Data Array"=w286) -> (w289:T5)
        n106 = call <vilib>:"Add State(s) to Queue__jki_lib_state_machine.vi"("State(s) in (\"\")"=w298) -> ("States Out"=w297:string)  [unwired: 14 in]
      }
      frame "Limits Test: Read Set" {
        w304 = "Read Set Test"  # Sub Test Name
        # "Equal to F1?"
        # "#Limits Testing - Add the sub test name for\ntest included in limits file"
        n107 = Unbundle By Name(w303) -> ("Results Data Array"=w301:string[][])
        n108 = Unbundle By Name(w303) -> ("Test Limits"=w305:string[][], "Read Set"=w309:string)
        n109 = To Variant(anything=w309) -> (Variant=w306:variant)
        n110 = call "Process Results.vi"("error in (no error)"=w307, "Measurement"=w306, "Test Limits"=w305, "Sub Test Name"=w304) -> ("error out"=w308:errorcluster, "Results Data"=w300:string[])  [unwired: 6 in]
        n111 = Build Array (concatenate)(w301, w300) -> (w299:string[][])
        n112 = Bundle By Name(cluster=w303, "Results Data Array"=w299) -> (w302:T5)
        n113 = call <vilib>:"Add State(s) to Queue__jki_lib_state_machine.vi"("State(s) in (\"\")"=w311) -> ("States Out"=w310:string)  [unwired: 14 in]
      }
      frame "Limits Test: Read Start" {
        w317 = "Read Start Test"  # Sub Test Name
        # "Equal to F1?"
        # "#Limits Testing - Add the sub test name for\ntest included in limits file"
        n114 = Unbundle By Name(w316) -> ("Results Data Array"=w314:string[][])
        n115 = Unbundle By Name(w316) -> ("Test Limits"=w318:string[][], "Read Start"=w322:string)
        n116 = To Variant(anything=w322) -> (Variant=w319:variant)
        n117 = call "Process Results.vi"("error in (no error)"=w320, "Measurement"=w319, "Test Limits"=w318, "Sub Test Name"=w317) -> ("error out"=w321:errorcluster, "Results Data"=w313:string[])  [unwired: 6 in]
        n118 = Build Array (concatenate)(w314, w313) -> (w312:string[][])
        n119 = Bundle By Name(cluster=w316, "Results Data Array"=w312) -> (w315:T5)
        n120 = call <vilib>:"Add State(s) to Queue__jki_lib_state_machine.vi"("State(s) in (\"\")"=w324) -> ("States Out"=w323:string)  [unwired: 14 in]
      }
      frame "Limits Test: eSTOP 1 Error Test" {
        w330 = "eSTOP 1 Error Test"  # Sub Test Name
        # "Equal to FF ?"
        # "#Limits Testing - Add the sub test name for\ntest included in limits file"
        n121 = Unbundle By Name(w329) -> ("Test Limits"=w331:string[][], "eSTOP 1 Error Test"=w335:string)
        n122 = Unbundle By Name(w329) -> ("Results Data Array"=w327:string[][])
        n123 = To Variant(anything=w335) -> (Variant=w332:variant)
        n124 = call "Process Results.vi"("error in (no error)"=w333, "Measurement"=w332, "Test Limits"=w331, "Sub Test Name"=w330) -> ("error out"=w334:errorcluster, "Results Data"=w326:string[])  [unwired: 6 in]
        n125 = Build Array (concatenate)(w327, w326) -> (w325:string[][])
        n126 = Bundle By Name(cluster=w329, "Results Data Array"=w325) -> (w328:T5)
        n127 = call <vilib>:"Add State(s) to Queue__jki_lib_state_machine.vi"("State(s) in (\"\")"=w337) -> ("States Out"=w336:string)  [unwired: 14 in]
      }
      frame "Limits Test: eSTOP 1 State Error Test" {
        w343 = "eSTOP 1 State Error Test"  # Sub Test Name
        # "Equal to FF ?"
        # "#Limits Testing - Add the sub test name for\ntest included in limits file"
        n128 = Unbundle By Name(w342) -> ("Test Limits"=w344:string[][], "eSTOP 1 State Error Test"=w348:string)
        n129 = Unbundle By Name(w342) -> ("Results Data Array"=w340:string[][])
        n130 = To Variant(anything=w348) -> (Variant=w345:variant)
        n131 = call "Process Results.vi"("error in (no error)"=w346, "Measurement"=w345, "Test Limits"=w344, "Sub Test Name"=w343) -> ("error out"=w347:errorcluster, "Results Data"=w339:string[])  [unwired: 6 in]
        n132 = Build Array (concatenate)(w340, w339) -> (w338:string[][])
        n133 = Bundle By Name(cluster=w342, "Results Data Array"=w338) -> (w341:T5)
        n134 = call <vilib>:"Add State(s) to Queue__jki_lib_state_machine.vi"("State(s) in (\"\")"=w350) -> ("States Out"=w349:string)  [unwired: 14 in]
      }
      frame "---------- Results Data ----------" {
        # "Template Separator\n(You can make a copy of, or modify, this frame)"
        n135 = call <vilib>:"Add State(s) to Queue__jki_lib_state_machine.vi"("State(s) in (\"\")"=w354) -> ("States Out"=w353:string)  [unwired: 14 in]
      }
      frame "Results Data: Write Results Data" {
        w356 = ","  # delimiter (\t)
        w357 = TRUE  # append to file? (new file:F)
        n136 = Unbundle By Name(w359) -> ("Results File Path"=w358:path, "Results Data Array"=w355:string[][])
        "Results Data Array" <- w355
        n137 = call-poly <vilib>:"Write Delimited Spreadsheet.vi"("file path (dialog if empty)"=w358, "2D data"=w355, "append to file? (new file:F)"=w357, "error in (no error)"=w360, "delimiter (\\t)"=w356) -> ("error out"=w361:errorcluster)  [unwired: 9 in, 1 out]
        n138 = call <vilib>:"Add State(s) to Queue__jki_lib_state_machine.vi"("State(s) in (\"\")"=w363) -> ("States Out"=w362:string)  [unwired: 14 in]
      }
      frame "---------- eSTOP1 Test ----------" {
        # "Template Separator\n(You can make a copy of, or modify, this frame)"
        n139 = call <vilib>:"Add State(s) to Queue__jki_lib_state_machine.vi"("State(s) in (\"\")"=w367) -> ("States Out"=w366:string)  [unwired: 14 in]
      }
      frame "eSTOP1 Test: Initialise" {
        # "Measurement initialisation code goes here"
        n140 = call "FGV - Initialise.vi"("Enum"=FGV_-_Enum."Get Data", "Error In"=w372) -> ("connection ID"=w369:refnum<k16>, "Handle Out"=w368:u64, "Error Out"=w371:errorcluster)  [unwired: 10 in, 1 out]
        n141 = Bundle By Name(cluster=w374, "connection ID"=w369, "handle out"=w368) -> (w373:T5)
        n142 = call <vilib>:"Add State(s) to Queue__jki_lib_state_machine.vi"("State(s) in (\"\")"=w376) -> ("States Out"=w375:string)  [unwired: 14 in]
      }
      frame "eSTOP1 Test: Set Command" {
        # "Data"
        # "Length"
        # "ID"
        # "Target"
        # "Type"
        # "Pkt ID"
        # "Measurement initialisation code goes here"
        n143 = Unbundle By Name(w394) -> ("connection ID"=w392:refnum<k16>)
        n144 = Build Array(u8 91 ("element"), u8 1 ("element"), u8 9 ("element"), u8 108 ("element"), u8 0 ("element")) -> (w386:u8[])
        n145 = String To IP(1:"192.168.201.21" ("name")) -> (0:w390:u32)
        n146 = Byte Array To String(unsigned byte array=w386) -> (string=w380:string)
        n147 = UDP Write(address=w390, port or service name=u16 54321, connection ID=w392, data in=w380, 8:w393, 9:1000 ("timeout ms (25000)")) -> (error out=w379:errorcluster, 3:w391:refnum<k16>)
        n148 = Bundle By Name(cluster=w394, "connection ID"=w391) -> (w395:T5)
        n149 = call <userlib>:"Wait (ms)__ogtk.vi"("error in (no error)"=w379, "milliseconds to wait"=u32 1000) -> ("error out"=w378:errorcluster)  [unwired: 8 in, 1 out]
        n150 = call <vilib>:"Add State(s) to Queue__jki_lib_state_machine.vi"("State(s) in (\"\")"=w397) -> ("States Out"=w396:string)  [unwired: 14 in]
      }
      frame "eSTOP1 Test: Read Set Command" {
        # "#56 = didnt read before the timeout"
        # "Measurement initialisation code goes here"
        n151 = Unbundle By Name(w406) -> ("connection ID"=w398:refnum<k16>)
        n152 = for {
          N: 1000 -> [_]
          shift-right: [w422] -> w401
          shift-left: w400 -> [w420]
          shift-right: [w421] -> w403
          shift-left: w398 -> [w424]
          tunnel: [w412] -> w402
          stop <- w410 stop-if-true
          n153 = UDP Read(connection ID=w424, timeout ms (25000)=1, 8:w420) -> (data out=w419:string, error out=w422:errorcluster, 3:w421:refnum<k16>)  [unwired: 1 in, 2 out]
          n154 = String Subset(string=w419, offset (0)=17 ("offset (0) 2"), length (rest)=1 ("length (rest) 2")) -> (substring=w418:string)
          n155 = String To Byte Array(string=w418) -> (unsigned byte array=w416:u8[])
          n156 = Number To Hexadecimal String(2:w416) -> (0:w417:string[])  [unwired: 1 in]
          n157 = Index Array(array=w417, index=0) -> (element=w412:string)
          n158 = Equal?(x=w412, y="15") -> (x = y?=w410:bool)
          "Wait for Start" <- w410
        }
        n159 = Bundle By Name(cluster=w406, "connection ID"=w403, "Read Set"=w402) -> (w407:T5)
        n160 = call <vilib>:"Clear Errors.vi"("error in (no error)"=w401, "specific error code to clear (0: all)"=56) -> ("error out"=w404:errorcluster)  [unwired: 4 in, 1 out]
        n161 = call <vilib>:"Add State(s) to Queue__jki_lib_state_machine.vi"("State(s) in (\"\")"=w409) -> ("States Out"=w408:string)  [unwired: 14 in]
      }
      frame "eSTOP1 Test: Start Command" {
        # "Data"
        # "Length"
        # "ID"
        # "Target"
        # "Type"
        # "Pkt ID"
        # "Measurement initialisation code goes here"
        n162 = Unbundle By Name(w442) -> ("connection ID"=w440:refnum<k16>)
        n163 = Build Array(u8 91 ("element"), u8 1 ("element"), u8 9 ("element"), u8 110 ("element"), u8 0 ("element")) -> (w434:u8[])
        n164 = String To IP(1:"192.168.201.21" ("name")) -> (0:w438:u32)
        n165 = Byte Array To String(unsigned byte array=w434) -> (string=w428:string)
        n166 = UDP Write(address=w438, port or service name=u16 54321, connection ID=w440, data in=w428, 8:w441, 9:1000 ("timeout ms (25000)")) -> (error out=w427:errorcluster, 3:w439:refnum<k16>)
        n167 = Bundle By Name(cluster=w442, "connection ID"=w439) -> (w443:T5)
        n168 = call <userlib>:"Wait (ms)__ogtk.vi"("error in (no error)"=w427, "milliseconds to wait"=u32 1000) -> ("error out"=w426:errorcluster)  [unwired: 8 in, 1 out]
        n169 = call <vilib>:"Add State(s) to Queue__jki_lib_state_machine.vi"("State(s) in (\"\")"=w445) -> ("States Out"=w444:string)  [unwired: 14 in]
      }
      frame "eSTOP1 Test: Read Start Command" {
        # "#56 = didnt read before the timeout"
        # "Measurement initialisation code goes here"
        n170 = Unbundle By Name(w454) -> ("connection ID"=w451:refnum<k16>)
        n171 = for {
          N: 1000 -> [_]
          shift-right: [w470] -> w447
          shift-left: w446 -> [w468]
          shift-right: [w469] -> w449
          shift-left: w451 -> [w472]
          tunnel: [w460] -> w448
          stop <- w458 stop-if-true
          n172 = UDP Read(connection ID=w472, timeout ms (25000)=1, 8:w468) -> (data out=w467:string, error out=w470:errorcluster, 3:w469:refnum<k16>)  [unwired: 1 in, 2 out]
          n173 = String Subset(string=w467, offset (0)=17 ("offset (0) 2"), length (rest)=1 ("length (rest) 2")) -> (substring=w466:string)
          n174 = String To Byte Array(string=w466) -> (unsigned byte array=w464:u8[])
          n175 = Number To Hexadecimal String(2:w464) -> (0:w465:string[])  [unwired: 1 in]
          n176 = Index Array(array=w465, index=0) -> (element=w460:string)
          n177 = Equal?(x=w460, y="19") -> (x = y?=w458:bool)
          "Normal Operation" <- w458
        }
        n178 = call <vilib>:"Clear Errors.vi"("error in (no error)"=w447, "specific error code to clear (0: all)"=56) -> ("error out"=w452:errorcluster)  [unwired: 4 in, 1 out]
        n179 = Bundle By Name(cluster=w454, "connection ID"=w449, "Read Start"=w448) -> (w455:T5)
        n180 = call <vilib>:"Add State(s) to Queue__jki_lib_state_machine.vi"("State(s) in (\"\")"=w457) -> ("States Out"=w456:string)  [unwired: 14 in]
      }
      frame "eSTOP1 Test: Start Timer" {
        # "Start Timer and slide bar"
        # "Template Separator\n(You can make a copy of, or modify, this frame)"
        n181 = call "Timer.vi"("error in (no error)"=w474, "Enum"=T4."Start Timer") -> ("error out"=w478:errorcluster)  [unwired: 6 in, 3 out]
        n182 = property on="Timeout - Test" class="Slide (strict)"(error in=w478, "Value"=0.0 ("Horizontal Pointer Slide"), "Scale.Maximum"=3.0 ("Target Time"), "Scale.Minimum"=0.0 ("Scale.Range:Minimum")) -> (error out=w473:errorcluster)  [unwired: 1 in, 1 out]
        n183 = call <vilib>:"Add State(s) to Queue__jki_lib_state_machine.vi"("State(s) in (\"\")"=w482) -> ("States Out"=w481:string)  [unwired: 14 in]
      }
      frame "eSTOP1 Test: I2C Measurment" {
        # "switch realy - trigger estop 1"
        n184 = Unbundle By Name(w485) -> ("handle out"=w487:u64)
        n185 = call "PCA9525 - Estop 1.vi"("error in (no error)"=w488, "buffer"=u8[] [2, 86, 0], "handle"=w487) -> ("error out"=w484:errorcluster, "handle out"=w486:u64)  [unwired: 6 in, 1 out]
        n186 = Bundle By Name(cluster=w485, "handle out"=w486) -> (w483:T5)
        n187 = call <vilib>:"Add State(s) to Queue__jki_lib_state_machine.vi"("State(s) in (\"\")"=w491) -> ("States Out"=w490:string)  [unwired: 14 in]
      }
      frame "eSTOP1 Test: UDP Read" {
        # "Read UDP if equal to F1 then test complete if false timer is check if elapsed"
        n188 = Unbundle By Name(w498) -> ("connection ID"=w507:refnum<k16>)
        n189 = UDP Read(connection ID=w507, timeout ms (25000)=10, 8:w499) -> (data out=w493:string, error out=w497:errorcluster, 3:w506:refnum<k16>)  [unwired: 1 in, 2 out]
        n190 = String Subset(string=w493, offset (0)=81 ("offset (0) 2"), length (rest)=1 ("length (rest) 2")) -> (substring=w505:string)
        n191 = String To Byte Array(string=w505) -> (unsigned byte array=w512:u8[])
        n192 = Number To Hexadecimal String(2:w512) -> (0:w511:string[])  [unwired: 1 in]
        n193 = Index Array(array=w511, index=0) -> (element=w501:string)
        n194 = Equal?(x=w501, y="F1") -> (x = y?=w492:bool)
        "eSTOP 1 Test" <- w492
        n195 = Bundle By Name(cluster=w498, "connection ID"=w506, "eSTOP 1 Test"=w501) -> (w513:T5)
        n196 = call <vilib>:"Clear Errors.vi"("error in (no error)"=w497, "specific error code to clear (0: all)"=56) -> ("error out"=w496:errorcluster)  [unwired: 4 in, 1 out]
        n197 = call-poly <vilib>:"Select State(s)__jki_lib_state_machine.vi"("State(s) if True (\"\")"="eSTOP1 Test: UDP Read (State)" ("State(s) if True (\"\")"), "Select"=w492, "State(s) if False (\"\")"="eSTOP1 Test: Elapsed Timer" ("State(s) if False (\"\")")) -> ("States Out"=w500:string)  [unwired: 12 in]
        n198 = call <vilib>:"Add State(s) to Queue__jki_lib_state_machine.vi"("State(s) in Front (\"\")"=w500, "State(s) in (\"\")"=w515) -> ("States Out"=w514:string)  [unwired: 13 in]
      }
      frame "eSTOP1 Test: UDP Read (State)" {
        # "Read UDP if equal to F1 then test complete if false timer is check if elapsed"
        n199 = Unbundle By Name(w522) -> ("connection ID"=w531:refnum<k16>)
        n200 = UDP Read(connection ID=w531, timeout ms (25000)=10, 8:w523) -> (data out=w517:string, error out=w521:errorcluster, 3:w530:refnum<k16>)  [unwired: 1 in, 2 out]
        n201 = String Subset(string=w517, offset (0)=17 ("offset (0) 2"), length (rest)=1 ("length (rest) 2")) -> (substring=w529:string)
        n202 = String To Byte Array(string=w529) -> (unsigned byte array=w536:u8[])
        n203 = Number To Hexadecimal String(2:w536) -> (0:w535:string[])  [unwired: 1 in]
        n204 = Index Array(array=w535, index=0) -> (element=w525:string)
        n205 = Equal?(x=w525, y="2") -> (x = y?=w516:bool)
        n206 = Bundle By Name(cluster=w522, "connection ID"=w530, "eSTOP 1 State Test"=w525) -> (w537:T5)
        n207 = call <vilib>:"Clear Errors.vi"("error in (no error)"=w521, "specific error code to clear (0: all)"=56) -> ("error out"=w520:errorcluster)  [unwired: 4 in, 1 out]
        n208 = call-poly <vilib>:"Select State(s)__jki_lib_state_machine.vi"("State(s) if True (\"\")"="Macro: Test (Error)" ("State(s) if True (\"\")"), "Select"=w516, "State(s) if False (\"\")"="eSTOP1 Test: Elapsed Timer" ("State(s) if False (\"\")")) -> ("States Out"=w524:string)  [unwired: 12 in]
        n209 = call <vilib>:"Add State(s) to Queue__jki_lib_state_machine.vi"("State(s) in Front (\"\")"=w524, "State(s) in (\"\")"=w539) -> ("States Out"=w538:string)  [unwired: 13 in]
      }
      frame "eSTOP1 Test: Elapsed Timer" {
        # "check if timer elapsed if true end of test if false UDP is read again,"
        # "Template Separator\n(You can make a copy of, or modify, this frame)"
        n210 = call "Timer.vi"("error in (no error)"=w544, "Target Time"=3.0, "Enum"=T4."Get Time") -> ("error out"=w543:errorcluster, "Time Elapsed?"=w545:bool, "Elapsed Time"=→"Timeout - Test":dbl)  [unwired: 5 in, 1 out]
        n211 = call-poly <vilib>:"Select State(s)__jki_lib_state_machine.vi"("State(s) if True (\"\")"="Macro: Test (Error)" ("State(s) if True (\"\")"), "Select"=w545, "State(s) if False (\"\")"="eSTOP1 Test: UDP Read" ("State(s) if False (\"\")")) -> ("States Out"=w542:string)  [unwired: 12 in]
        n212 = call <vilib>:"Add State(s) to Queue__jki_lib_state_machine.vi"("State(s) in Front (\"\")"=w542, "State(s) in (\"\")"=w551) -> ("States Out"=w550:string)  [unwired: 13 in]
      }
      frame "eSTOP1 Test: Reset" {
        # "Switch relays - back to Initialize state"
        # "Measurment cleanup code goes here"
        n213 = Unbundle By Name(w553) -> ("handle out"=w557:u64)
        n214 = call "PCA9525 - Estop 1.vi"("error in (no error)"=w554, "buffer"=u8[] [2, 85, 0], "handle"=w557) -> ("error out"=w555:errorcluster, "handle out"=w556:u64)  [unwired: 6 in, 1 out]
        n215 = Bundle By Name(cluster=w553, "handle out"=w556) -> (w552:T5)
        n216 = call <vilib>:"Add State(s) to Queue__jki_lib_state_machine.vi"("State(s) in (\"\")"=w560) -> ("States Out"=w559:string)  [unwired: 14 in]
      }
      frame "eSTOP1 Test: Set Command (Error)" {
        # "Data"
        # "Length"
        # "ID"
        # "Target"
        # "Type"
        # "Pkt ID"
        # "Measurement initialisation code goes here"
        n217 = Unbundle By Name(w579) -> ("connection ID"=w577:refnum<k16>)
        n218 = Build Array(u8 91 ("element"), u8 1 ("element"), u8 9 ("element"), u8 108 ("element"), u8 0 ("element")) -> (w571:u8[])
        n219 = String To IP(1:"192.168.201.21" ("name")) -> (0:w575:u32)
        n220 = Byte Array To String(unsigned byte array=w571) -> (string=w565:string)
        n221 = UDP Write(address=w575, port or service name=u16 54321, connection ID=w577, data in=w565, 8:w578, 9:1000 ("timeout ms (25000)")) -> (error out=w564:errorcluster, 3:w576:refnum<k16>)
        n222 = Bundle By Name(cluster=w579, "connection ID"=w576) -> (w580:T5)
        n223 = call <userlib>:"Wait (ms)__ogtk.vi"("error in (no error)"=w564, "milliseconds to wait"=u32 20000) -> ("error out"=w563:errorcluster, "millisecond timer value"=→"Wait - Reset":u32)  [unwired: 8 in]
        n224 = call <vilib>:"Add State(s) to Queue__jki_lib_state_machine.vi"("State(s) in (\"\")"=w582) -> ("States Out"=w581:string)  [unwired: 14 in]
      }
      frame "eSTOP1 Test: Start Command (Error)" {
        # "Data"
        # "Length"
        # "ID"
        # "Target"
        # "Type"
        # "Pkt ID"
        # "Measurement initialisation code goes here"
        n225 = Unbundle By Name(w600) -> ("connection ID"=w598:refnum<k16>)
        n226 = Build Array(u8 91 ("element"), u8 1 ("element"), u8 9 ("element"), u8 110 ("element"), u8 0 ("element")) -> (w592:u8[])
        n227 = String To IP(1:"192.168.201.21" ("name")) -> (0:w596:u32)
        n228 = Byte Array To String(unsigned byte array=w592) -> (string=w586:string)
        n229 = UDP Write(address=w596, port or service name=u16 54321, connection ID=w598, data in=w586, 8:w599, 9:1000 ("timeout ms (25000)")) -> (error out=w585:errorcluster, 3:w597:refnum<k16>)
        n230 = Bundle By Name(cluster=w600, "connection ID"=w597) -> (w601:T5)
        n231 = call <userlib>:"Wait (ms)__ogtk.vi"("error in (no error)"=w585, "milliseconds to wait"=u32 5000) -> ("error out"=w584:errorcluster)  [unwired: 8 in, 1 out]
        n232 = call <vilib>:"Add State(s) to Queue__jki_lib_state_machine.vi"("State(s) in (\"\")"=w603) -> ("States Out"=w602:string)  [unwired: 14 in]
      }
      frame "eSTOP1 Test: Start Timer (Error)" {
        # "Template Separator\n(You can make a copy of, or modify, this frame)"
        n233 = call "Timer.vi"("error in (no error)"=w606, "Enum"=T4."Start Timer") -> ("error out"=w610:errorcluster)  [unwired: 6 in, 3 out]
        n234 = property on="Timeout - Error Test" class="Slide (strict)"(error in=w610, "Value"=0.0 ("Horizontal Pointer Slide"), "Scale.Maximum"=3.0 ("Target Time"), "Scale.Minimum"=0.0 ("Scale.Range:Minimum")) -> (error out=w605:errorcluster)  [unwired: 1 in, 1 out]
        n235 = call <vilib>:"Add State(s) to Queue__jki_lib_state_machine.vi"("State(s) in Front (\"\")"="eSTOP1 Test: I2C Error Measurment" ("State(s) if True (\"\")"), "State(s) in (\"\")"=w614) -> ("States Out"=w613:string)  [unwired: 13 in]
      }
      frame "eSTOP1 Test: I2C Error Measurment" {
        # "switch relay - force error"
        n236 = Unbundle By Name(w618) -> ("handle out"=w620:u64)
        n237 = call "PCA9525 - Estop 1.vi"("error in (no error)"=w621, "buffer"=u8[] [2, 3, 0], "handle"=w620) -> ("error out"=w617:errorcluster, "handle out"=w619:u64)  [unwired: 6 in, 1 out]
        n238 = Bundle By Name(cluster=w618, "handle out"=w619) -> (w616:T5)
        n239 = call <vilib>:"Add State(s) to Queue__jki_lib_state_machine.vi"("State(s) in Front (\"\")"="eSTOP1 Test: Error UDP Read" ("State(s) if True (\"\")"), "State(s) in (\"\")"=w624) -> ("States Out"=w623:string)  [unwired: 13 in]
      }
      frame "eSTOP1 Test: Error UDP Read" {
        # "Read UDP if equal to FF test complete if false check if timer has elapsed."
        n240 = Unbundle By Name(w631) -> ("connection ID"=w642:refnum<k16>)
        n241 = UDP Read(connection ID=w642, timeout ms (25000)=100, 8:w632) -> (data out=w645:string, error out=w630:errorcluster, 3:w641:refnum<k16>)  [unwired: 1 in, 2 out]
        n242 = String Subset(string=w645, offset (0)=81 ("offset (0) 2"), length (rest)=1 ("length (rest) 2")) -> (substring=w626:string)
        n243 = String To Byte Array(string=w626) -> (unsigned byte array=w640:u8[])
        n244 = Number To Hexadecimal String(2:w640) -> (0:w639:string[])  [unwired: 1 in]
        n245 = Index Array(array=w639, index=0) -> (element=w634:string)
        n246 = Bundle By Name(cluster=w631, "connection ID"=w641, "eSTOP 1 Error Test"=w634) -> (w646:T5)
        n247 = Equal?(x=w634, y="FF") -> (x = y?=w625:bool)
        "eSTOP 1 Error Test" <- w625
        n248 = call <vilib>:"Clear Errors.vi"("error in (no error)"=w630, "specific error code to clear (0: all)"=56) -> ("error out"=w629:errorcluster)  [unwired: 4 in, 1 out]
        n249 = call-poly <vilib>:"Select State(s)__jki_lib_state_machine.vi"("State(s) if True (\"\")"="eSTOP1 Test: Error UDP Read (State)" ("State(s) if True (\"\")"), "Select"=w625, "State(s) if False (\"\")"="eSTOP1 Test: Elapsed Timer (Error)" ("State(s) if False (\"\")")) -> ("States Out"=w633:string)  [unwired: 12 in]
        n250 = call <vilib>:"Add State(s) to Queue__jki_lib_state_machine.vi"("State(s) in Front (\"\")"=w633, "State(s) in (\"\")"=w648) -> ("States Out"=w647:string)  [unwired: 13 in]
      }
      frame "eSTOP1 Test: Error UDP Read (State)" {
        # "Read UDP if equal to FF test complete if false check if timer has elapsed."
        n251 = Unbundle By Name(w655) -> ("connection ID"=w666:refnum<k16>)
        n252 = UDP Read(connection ID=w666, timeout ms (25000)=100, 8:w656) -> (data out=w669:string, error out=w654:errorcluster, 3:w665:refnum<k16>)  [unwired: 1 in, 2 out]
        n253 = String Subset(string=w669, offset (0)=17 ("offset (0) 2"), length (rest)=1 ("length (rest) 2")) -> (substring=w650:string)
        n254 = String To Byte Array(string=w650) -> (unsigned byte array=w664:u8[])
        n255 = Number To Hexadecimal String(2:w664) -> (0:w663:string[])  [unwired: 1 in]
        n256 = Index Array(array=w663, index=0) -> (element=w658:string)
        n257 = Bundle By Name(cluster=w655, "connection ID"=w665, "eSTOP 1 State Error Test"=w658) -> (w670:T5)
        n258 = Equal?(x=w658, y="2") -> (x = y?=w649:bool)
        n259 = call <vilib>:"Clear Errors.vi"("error in (no error)"=w654, "specific error code to clear (0: all)"=56) -> ("error out"=w653:errorcluster)  [unwired: 4 in, 1 out]
        n260 = call-poly <vilib>:"Select State(s)__jki_lib_state_machine.vi"("State(s) if True (\"\")"="Macro: Limits" ("State(s) if True (\"\")"), "Select"=w649, "State(s) if False (\"\")"="eSTOP1 Test: Elapsed Timer (Error)" ("State(s) if False (\"\")")) -> ("States Out"=w657:string)  [unwired: 12 in]
        n261 = call <vilib>:"Add State(s) to Queue__jki_lib_state_machine.vi"("State(s) in Front (\"\")"=w657, "State(s) in (\"\")"=w672) -> ("States Out"=w671:string)  [unwired: 13 in]
      }
      frame "eSTOP1 Test: Elapsed Timer (Error)" {
        # "check if timer elapsed if true end of test if false UDP is read again,"
        # "Template Separator\n(You can make a copy of, or modify, this frame)"
        n262 = call "Timer.vi"("error in (no error)"=w677, "Target Time"=3.0, "Enum"=T4."Get Time") -> ("error out"=w676:errorcluster, "Time Elapsed?"=w678:bool, "Elapsed Time"=→"Timeout - Error Test":dbl)  [unwired: 5 in, 1 out]
        n263 = call-poly <vilib>:"Select State(s)__jki_lib_state_machine.vi"("State(s) if True (\"\")"="Macro: Limits" ("State(s) if True (\"\")"), "Select"=w678, "State(s) if False (\"\")"="eSTOP1 Test: Error UDP Read" ("State(s) if False (\"\")")) -> ("States Out"=w675:string)  [unwired: 12 in]
        n264 = call <vilib>:"Add State(s) to Queue__jki_lib_state_machine.vi"("State(s) in Front (\"\")"=w675, "State(s) in (\"\")"=w684) -> ("States Out"=w683:string)  [unwired: 13 in]
      }
      frame "eSTOP1 Test: Cleanup" {
        # "Switch relays - back to Initialize state"
        # "Measurment cleanup code goes here"
        n265 = Unbundle By Name(w686) -> ("handle out"=w690:u64)
        n266 = call "PCA9525 - Estop 1.vi"("error in (no error)"=w687, "buffer"=u8[] [2, 85, 0], "handle"=w690) -> ("error out"=w688:errorcluster, "handle out"=w689:u64)  [unwired: 6 in, 1 out]
        n267 = Bundle By Name(cluster=w686, "handle out"=w689) -> (w685:T5)
        n268 = call <vilib>:"Add State(s) to Queue__jki_lib_state_machine.vi"("State(s) in (\"\")"=w693) -> ("States Out"=w692:string)  [unwired: 14 in]
      }
    }
    n269 = Wait (ms)(milliseconds to wait=u32 1) -> ()  [unwired: 1 out]
  }
  "error out" <- w1
